vi "bool to msgpack.vi"(11 "Boolean":bool=TRUE) -> (3 "msgpack":u8[](array[numeric]) format="%x")   [LabVIEW 2020, in "MessagePack.lvlib" / "MessagePack.lvclass"]
uses:
  MessagePack.lvclass
  MessagePack.lvclass/MessagePack.ctl
  MsgPack Object Types.ctl
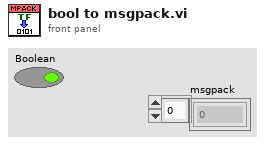
[diagram p1: front panel]
types:
  T1 = typedef "MessagePack.lvlib/MessagePack.lvclass/MsgPack Object Types.ctl" = enum16{"UNSUPPORTED", "POSINT", "NEGINT", "FIXMAP", "FIXARRAY", "FIXSTR", "NIL", "FALSE", "TRUE", "BIN8", "BIN16", "BIN32", "EXT8", "EXT16", "EXT32", "FLOAT32", "FLOAT64", "UINT8", "UINT16", "UINT32", "UINT64", "INT8", "INT16", "INT32", "INT64", "FIXEXT1", "FIXEXT2", "FIXEXT4", "FIXEXT8", "FIXEXT16", "STR8", "STR16", "STR32", "ARRAY16", "ARRAY32", "MAP16", "MAP32"}
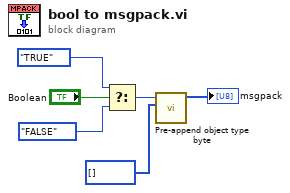
[diagram p0: block diagram]
diagram:
  n1 = Select(t=MsgPack_Object_Types."TRUE" ("MsgPack Object Type"), s="Boolean", f=MsgPack_Object_Types."FALSE" ("MsgPack Object Type")) -> (s? t:f=w3:T1)
  n2 = call "Pre-append object type byte.vi"("bytes in"=u8[] [], "Object type"=w3) -> ("encoded bytes"=→"msgpack":u8[])  [unwired: 8 in, 1 out]
